vi "DFT_normalizada.vi"(9 "FFT size":i32, 10 "X[n]":dbl[](array[numeric]), 11 "WaveformGraph in":refnum<vi>) -> (4 "DFTnorm":cdb[](array[numeric]))   [LabVIEW 2020]
uses:
  <vilib>/Analysis/2dsp.llb/Real FFT.vi
  <vilib>/Analysis/NI_AALPro.lvlib
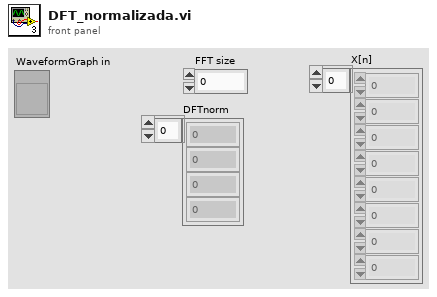
[diagram p1: front panel]
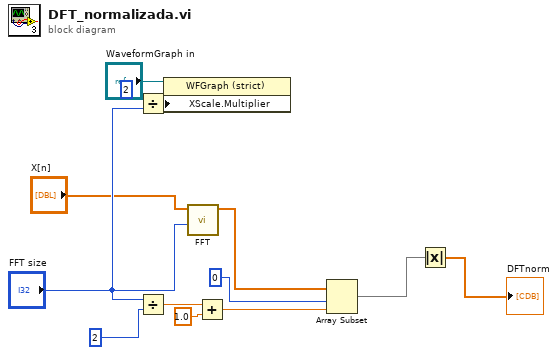
[diagram p0: block diagram]
diagram:
  n1 = Divide(x=2, y="FFT size") -> (x/y=w13:dbl)
  n2 = Divide(x="FFT size", y=2) -> (x/y=w10:dbl)
  n3 = property on="Property Node" class="WFGraph (strict)"(reference="WaveformGraph in", "XScale.Multiplier"=w13) -> ()  [unwired: 1 in, 2 out]
  n4 = call-poly <vilib>:"FFT.vi"("FFT size"="FFT size", "X"="X[n]") -> ("FFT {X}"=w12:cdb[])  [unwired: 8 in, 1 out]
  n5 = Add(x=w10, y=1.0) -> (x+y=w11:dbl)
  n6 = Array Subset(array=w12, index=0, length=w11) -> (w2:cdb[])
  n7 = Absolute Value(x=w2) -> (abs(x)=→"DFTnorm":dbl[])
